vi "Int16 Create.vi"(8 "error in (no error)":errorcluster, 11 "I16 in":i16) -> (0 "error out":errorcluster, 3 "Int16 DVR out":refnum<data-value>)   [LabVIEW 2012, in "MDSplus.lvlib"]
uses:
  <vilib>/MDSplus/Library/MDSplus.lvlib
  <vilib>/MDSplus/Classes/Data_Class/Scalar_Class/Int16_Class/Int16.lvclass
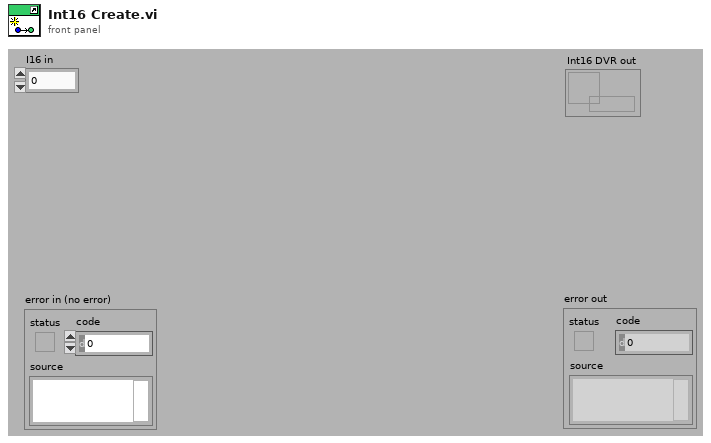
[diagram p1: front panel]
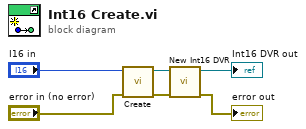
[diagram p0: block diagram]
diagram:
  n1 = call <vilib>:"Create.vi"("error in (no error)"="error in (no error)", "I16 in"="I16 in") -> ("error out"=w3:errorcluster, "Int16 out"=w4:refnum<class "Int16.lvclass">)  [unwired: 8 in]
  n2 = call <vilib>:"New Int16 DVR.vi"("error in (no error)"=w3, "Int16 in"=w4) -> ("error out"=→"error out":errorcluster, "Int16 DVR out"=→"Int16 DVR out":refnum<data-value>)  [unwired: 8 in]
